vi "Exemple_guider_3_1.vi"() -> ()   [LabVIEW 2018]
panel:
  out "Produit":u16
  out "N-2":u8
  out "N-1":u8
  out "N":u8
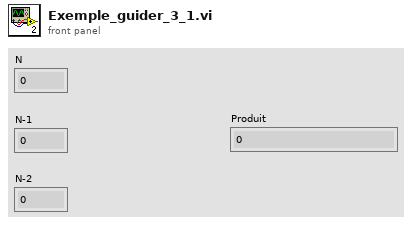
[diagram p1: front panel]
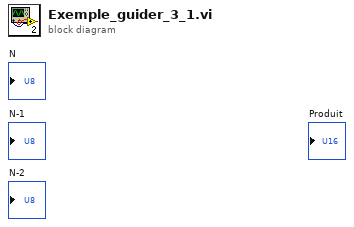
[diagram p0: block diagram]
diagram:
